vi "GOOD_Rev_01.vi"(10 "Input Data":dbl[](array[numeric]), 11 "Mean In":dbl=1600.0) -> (3 "GOOD":bool)   [LabVIEW 2012]
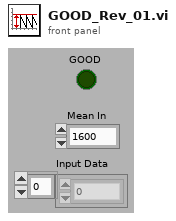
[diagram p1: front panel]
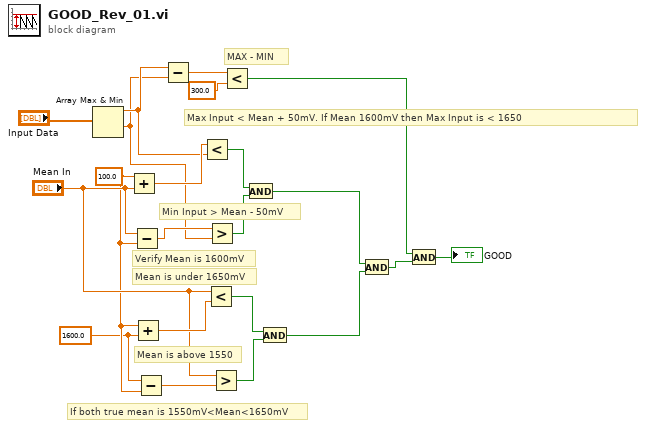
[diagram p0: block diagram]
diagram:
  w16 = 1600.0
  w17 = 100.0
  # "MAX - MIN"
  # "Min Input > Mean - 50mV"
  # "Max Input < Mean + 50mV. If Mean 1600mV then Max Input is < 1650"
  # "If both true mean is 1550mV<Mean<1650mV"
  # "Mean is above 1550"
  # "Mean is under 1650mV"
  # "Verify Mean is 1600mV"
  n1 = Array Max & Min(array="Input Data") -> (max value=w8:dbl, min value=w7:dbl)  [unwired: 2 out]
  n2 = Add(x=w17, y="Mean In") -> (x+y=w10:dbl)
  n3 = Subtract(x="Mean In", y=w17) -> (x-y=w9:dbl)
  n4 = Add(x=w17, y=w16) -> (x+y=w20:dbl)
  n5 = Subtract(x=w16, y=w17) -> (x-y=w19:dbl)
  n6 = Subtract(x=w8, y=w7) -> (x-y=w6:dbl)
  n7 = Less?(x=w10, y=w8) -> (x < y?=w15:bool)
  n8 = Less?(x="Mean In", y=w20) -> (x < y?=w13:bool)
  n9 = Greater?(x=w9, y=w7) -> (0:w14:bool)
  n10 = Greater?(x="Mean In", y=w19) -> (0:w12:bool)
  n11 = Less?(x=w6, y=300.0) -> (x < y?=w2:bool)
  n12 = And(x=w15, y=w14) -> (x .and. y?=w4:bool)
  n13 = And(x=w13, y=w12) -> (x .and. y?=w11:bool)
  n14 = And(x=w4, y=w11) -> (x .and. y?=w3:bool)
  n15 = And(x=w2, y=w3) -> (x .and. y?=→"GOOD":bool)
